vi "Mutex Timed Lock (relative seconds).vi"(8 "error in (no error)":errorcluster, 10 "relative timeout (seconds)":dbl, 11 "Mutex in":T1) -> (0 "error out":errorcluster, 2 "timed out?":bool, 3 "Mutex out":T1)   [LabVIEW 2013, in "POSIX Threads.lvlib" / "Mutex.lvclass"]
uses:
  Mutex.lvclass
  Controls/reference.ctl
  <vilib>/NI/NI Linux RT Utilities/Controls/Public/C Enums/clockid_t.ctl
  POSIX Thread Object/POSIX Thread Object.lvclass/POSIX Thread Object.ctl
  POSIX Thread Object/Private VIs/libpthread path.vi
  <vilib>/NI/NI Linux RT Utilities/VIs/Public/Convert Types/convert timespec 64 to timespec 32.vi
  <vilib>/NI/NI Linux RT Utilities/VIs/Public/Time/Increment Time (timespec).vi
  <vilib>/NI/NI Linux RT Utilities/VIs/Public/Time/Get Clock Time (timespec).vi
  POSIX Thread Object/Private VIs/get pthread error.vi
  POSIX Thread Object/POSIX Thread Object.lvclass
  <vilib>/NI/NI Linux RT Utilities/Linux RT Utilities.lvlib
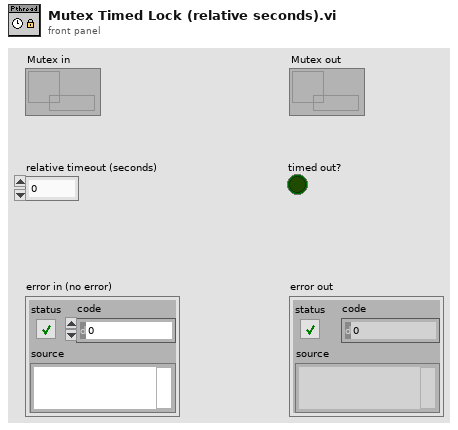
[diagram p1: front panel]
types:
  T1 = typedef "POSIX Threads.lvlib/Mutex.lvclass/reference.ctl" = refnum<data-value>
  T2 = typedef "Linux RT Utilities.lvlib/clockid_t.ctl" = enum16{"Realtime", "Monotonic"}
  T3 = typedef "Linux RT Utilities.lvlib/timespec_64.ctl" = cluster{"sec":u64, "nsec":u64}
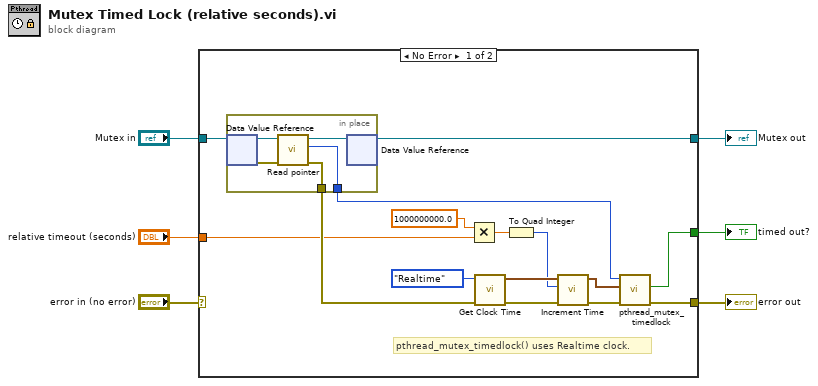
[diagram p0: block diagram]
diagram:
  n1 = case shown="No Error" "error in (no error)" {
    selector: "error in (no error)" -> [_ w28]
    tunnel: [w21 w28] -> w5
    tunnel: "Mutex in" -> [w11 w27]
    tunnel: [w7 w27] -> w3
    tunnel: "relative timeout (seconds)" -> [w9 _]
    tunnel: [w20 _] -> w1
    frame No Error {
      # "pthread_mutex_timedlock() uses Realtime clock."
      n2 = in-place {
        in-place-border: [w23] -> w10
        in-place-border: [w22] -> w8
        n3 = in-place-dvr #1(w11) -> (w26:refnum<class "Mutex.lvclass">, w24:errorcluster)
        n4 = call "Read pointer.vi"("error in (no error)"=w24, "POSIX Thread Object in"=w26) -> ("error out"=w23:errorcluster, "pointer"=w22:u64, "POSIX Thread Object out"=w25:refnum<class "Mutex.lvclass">)  [unwired: 7 in]
        n5 = in-place-dvr #1(w25) -> (w7:T1)  [unwired: 1 out]
      }
      n6 = Multiply(x=1000000000.0, y=w9) -> (x*y=w15:dbl)
      n7 = call-poly <vilib>:"Get Clock Time.vi"("error in (no error)"=w10, "clock id (monotonic)"=clockid_t."Realtime") -> ("error out"=w17:errorcluster, "timespec"=w18:T3)  [unwired: 8 in]
      n8 = To Quad Integer(1:w15) -> (0:w14:i64)
      n9 = call-poly <vilib>:"Increment Time.vi"("error in (no error)"=w17, "nanoseconds"=w14, "timespec in"=w18) -> ("error out"=w12:errorcluster, "timespec out"=w13:T3)  [unwired: 7 in]
      n10 = call "pthread_mutex_timedlock.vi"("error in (no error)"=w12, "absolute time"=w13, "mutex ptr in"=w8) -> ("error out"=w21:errorcluster, "timed out?"=w20:bool)  [unwired: 6 in, 1 out]
    }
    frame Error {
    }
  }
  "Mutex out" <- w3
  "error out" <- w5
  "timed out?" <- w1
